vi "Ball-Color.vi"() -> ()   [LabVIEW 2019]
uses:
  <vilib>/Rock Robotics/SystemInterfaces/i2clib/i2c_bus.ctl
  Robot Global Data.vi
panel:
  in  "Other":cluster{"R":dbl, "G":dbl, "B":dbl}={"R"=0.361, "G"=0.524, "B"=0.113}
  out "See":bool
  in  "Blue Calibration":cluster{"R":dbl, "G":dbl, "B":dbl}={"R"=0.143, "G"=0.427, "B"=0.429}
  in  "Green Calibration":cluster{"R":dbl, "G":dbl, "B":dbl}={"R"=0.197, "G"=0.561, "B"=0.24}
  in  "Red Calibration":cluster{"R":dbl, "G":dbl, "B":dbl}={"R"=0.561, "G"=0.323, "B"=0.114}
  in  "Yellow Calibration":cluster{"R":dbl, "G":dbl, "B":dbl}={"R"=0.361, "G"=0.524, "B"=0.113}
  in  "I2C Bus":T1
  out "Color":u32(colorbox)
  out "Proximity":u16(graph)
  out "error out":errorcluster
  out "Measured Color":cluster{"R":dbl, "G":dbl, "B":dbl}
  out "Match Confidence":dbl
  out "Matched Color Name":string
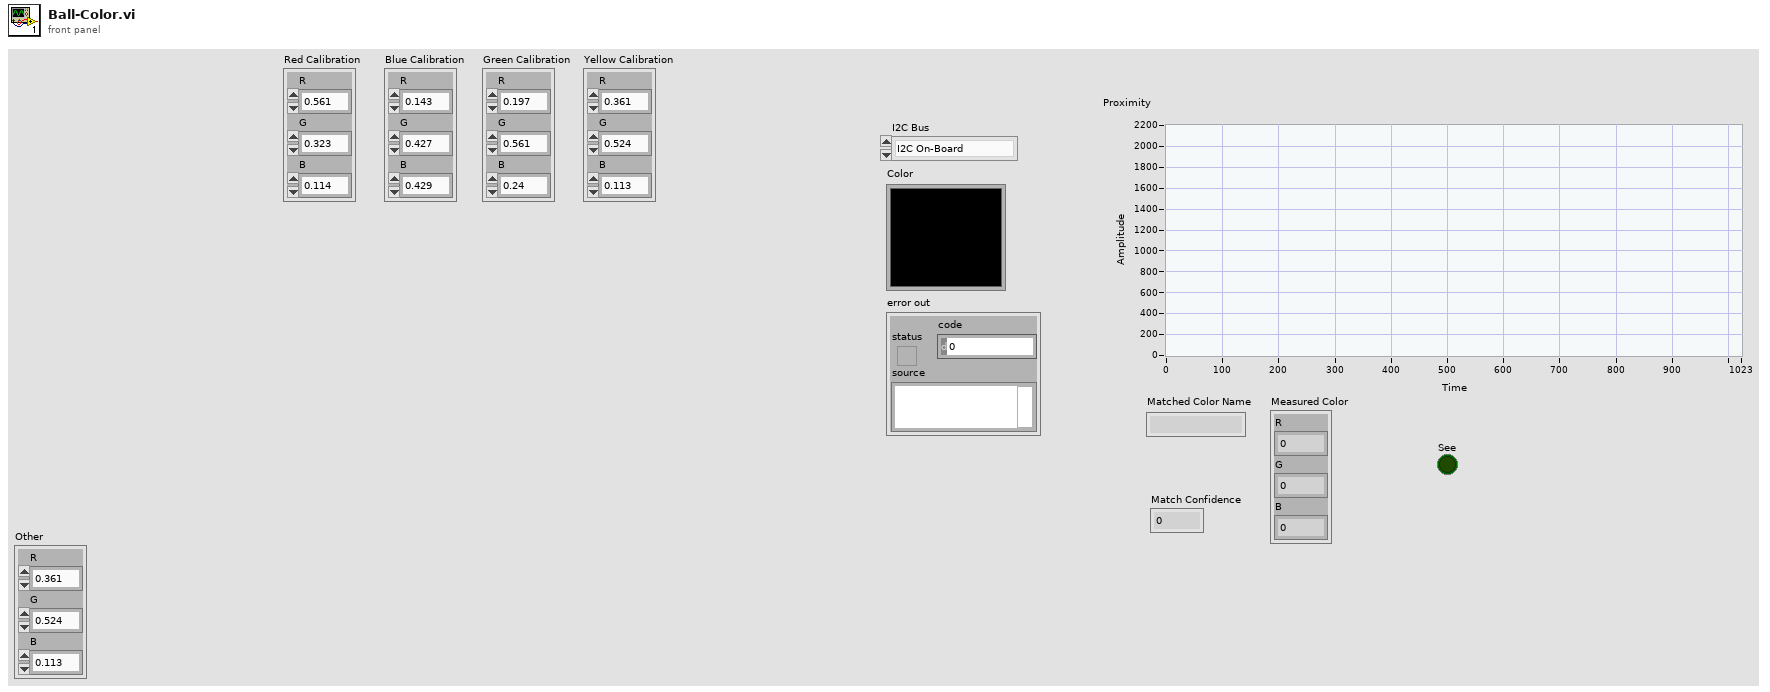
[diagram p1: front panel]
types:
  T1 = typedef "i2c_bus.ctl" = enum16{"I2C On-Board", "I2C MXP", "Invalid"}
  T2 = typedef "Color Sensor V3 DevRef.ctl" = cluster{"I2CDevRef":T3}
  T3 = typedef "WPI_I2CDevRef.ctl" = cluster{"DevStatus":errorcluster, "Device Address":u8, "Handle":i32, "I2C Bus":T1}
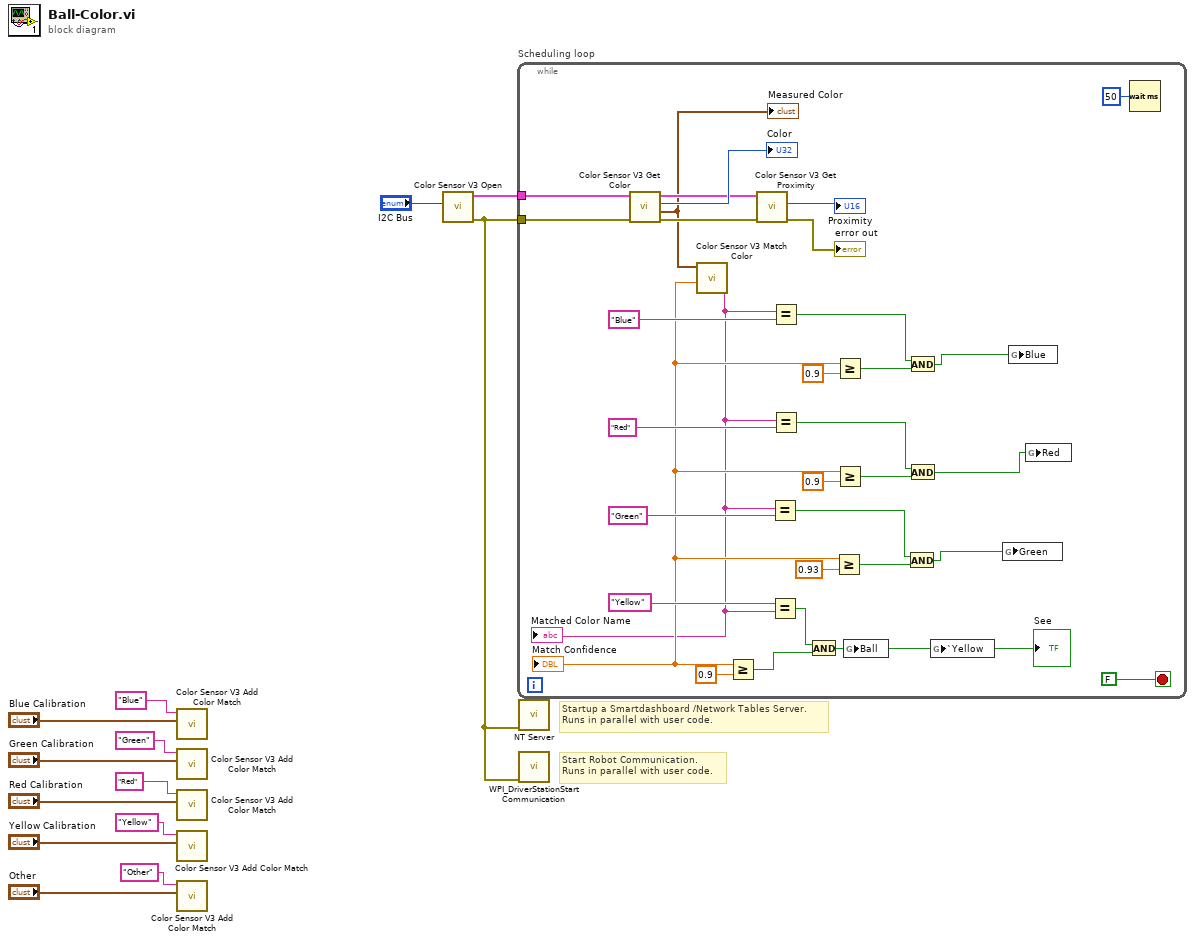
[diagram p0: block diagram]
diagram:
  # "Startup a Smartdashboard /Network Tables Server.\nRuns in parallel with user code."
  # "Start Robot Communication.\nRuns in parallel with user code."
  n1 = call <vilib>:"Color Sensor V3 Add Color Match.vi"("Color"="Blue Calibration", "Name"="Blue") -> ()  [unwired: 10 in]
  n2 = call <vilib>:"Color Sensor V3 Add Color Match.vi"("Color"="Green Calibration", "Name"="Green") -> ()  [unwired: 10 in]
  n3 = call <vilib>:"Color Sensor V3 Add Color Match.vi"("Color"="Red Calibration", "Name"="Red") -> ()  [unwired: 10 in]
  n4 = call <vilib>:"Color Sensor V3 Add Color Match.vi"("Color"="Yellow Calibration", "Name"="Yellow") -> ()  [unwired: 10 in]
  n5 = call <vilib>:"Color Sensor V3 Add Color Match.vi"("Color"="Other", "Name"="Other") -> ()  [unwired: 10 in]
  n6 = call <vilib>:"Color Sensor V3 Open.vi"("I2C Bus"="I2C Bus") -> ("error out"=w11:errorcluster, "ColorSensorDevRef"=w12:T2)  [unwired: 9 in]
  n7 = while "Scheduling loop" {
    tunnel: w12 -> [w39]
    tunnel: w11 -> [w38]
    stop <- FALSE stop-if-true
    n8 = call <vilib>:"Color Sensor V3 Get Color.vi"("error in (no error)"=w38, "ColorSensorDevRef"=w39) -> ("error out"=w43:errorcluster, "Normalized Color"=w37:cluster{"R":dbl, "G":dbl, "B":dbl}, "Color"=→"Color":u32, "ColorSensorDevRef out"=w42:T2)  [unwired: 6 in]
    "Measured Color" <- w37
    n9 = call <vilib>:"Color Sensor V3 Match Color.vi"("Measured Color"=w37) -> ("Confidence"=w22:dbl, "Matched Color Name"=w21:string)  [unwired: 8 in, 1 out]
    "Match Confidence" <- w22
    "Matched Color Name" <- w21
    n10 = Greater Or Equal?(x=w22, y=0.9) -> (x >= y?=w33:bool)
    n11 = call <vilib>:"Color Sensor V3 Get Proximity.vi"("error in (no error)"=w43, "ColorSensorDevRef"=w42) -> ("error out"=→"error out":errorcluster, "Proximity"=→"Proximity":u16)  [unwired: 7 in, 1 out]
    n12 = Equal?(x=w21, y="Green" ("Matched Color Name")) -> (x = y?=w14:bool)
    n13 = Equal?(x="Yellow", y=w21) -> (x = y?=w30:bool)
    n14 = Equal?(x=w21, y="Blue" ("Matched Color Name")) -> (x = y?=w20:bool)
    n15 = Equal?(x=w21, y="Red" ("Matched Color Name")) -> (x = y?=w17:bool)
    n16 = And(x=w30, y=w33) -> (x .and. y?=w31:bool)
    "See" <- w31
    n17 = Greater Or Equal?(x=w22, y=0.93) -> (x >= y?=w15:bool)
    n18 = Greater Or Equal?(x=w22, y=0.9) -> (x >= y?=w23:bool)
    n19 = Greater Or Equal?(x=w22, y=0.9) -> (x >= y?=w27:bool)
    n20 = global write "Robot Global Data.vi" "Ball"(w31) -> ()
    n21 = And(x=w14, y=w15) -> (x .and. y?=w16:bool)
    n22 = And(x=w20, y=w23) -> (x .and. y?=w19:bool)
    n23 = And(x=w17, y=w27) -> (x .and. y?=w18:bool)
    n24 = global write "Robot Global Data.vi" "`Yellow"(w31) -> ()
    n25 = global write "Robot Global Data.vi" "Green"(w16) -> ()
    n26 = global write "Robot Global Data.vi" "Blue"(w19) -> ()
    n27 = global write "Robot Global Data.vi" "Red"(w18) -> ()
    n28 = Wait (ms)(milliseconds to wait=u32 50) -> ()  [unwired: 1 out]
  }
  n29 = call <vilib>:"NT Server.vi"("error in (no error)"=w11) -> ()  [unwired: 11 in]
  n30 = call <vilib>:"WPI_DriverStationStart Communication.vi"("error in (no error)"=w11) -> ()  [unwired: 1 in, 10 out]
